vi "sub_tcp_fgv.vi"(7 "cmd":enum16{"ini", "read", "write", "close"}(ring), 8 "error in (no error)":errorcluster caption="error in", 11 "write_data":string) -> (0 "error out":errorcluster, 2 "data_check":bool, 3 "read_data":string)   [LabVIEW 2018]
panel:
  out "byte":u8[](array[numeric])
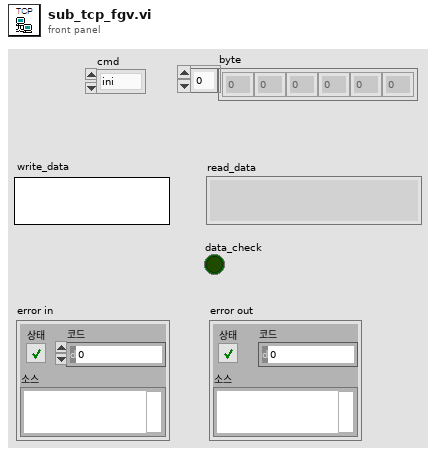
[diagram p1: front panel]
types:
  T1 = enum16{"Standard", "Buffered", "CRLF", "Immediate"}
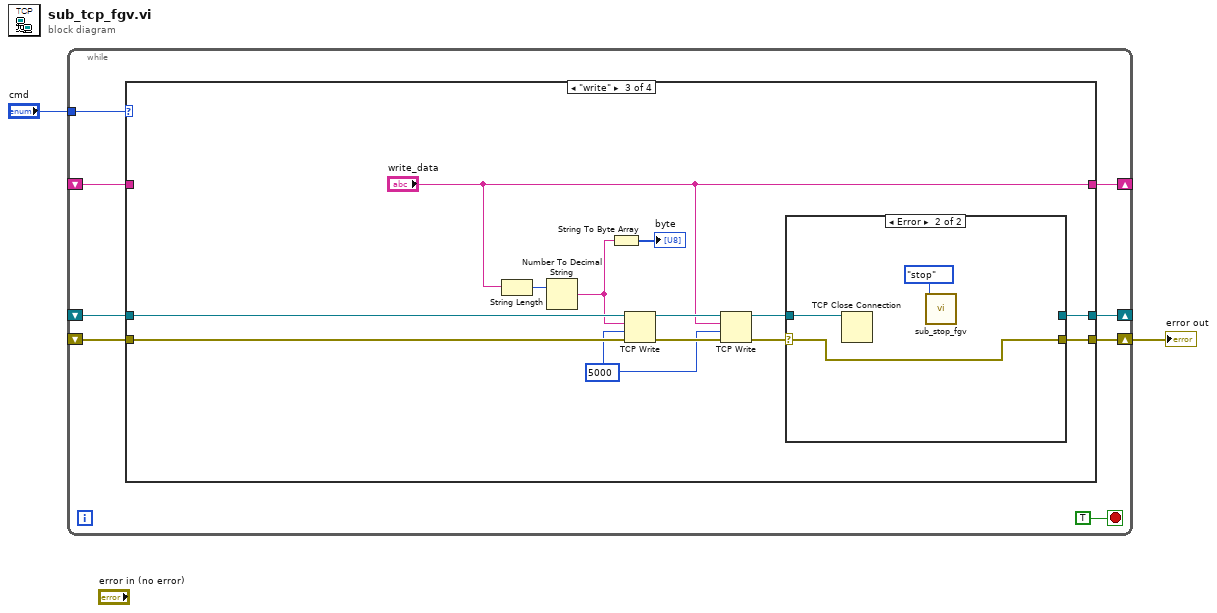
[diagram p0: block diagram]
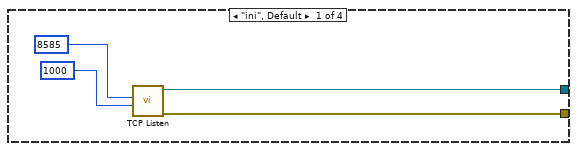
[diagram p2: hidden frame]
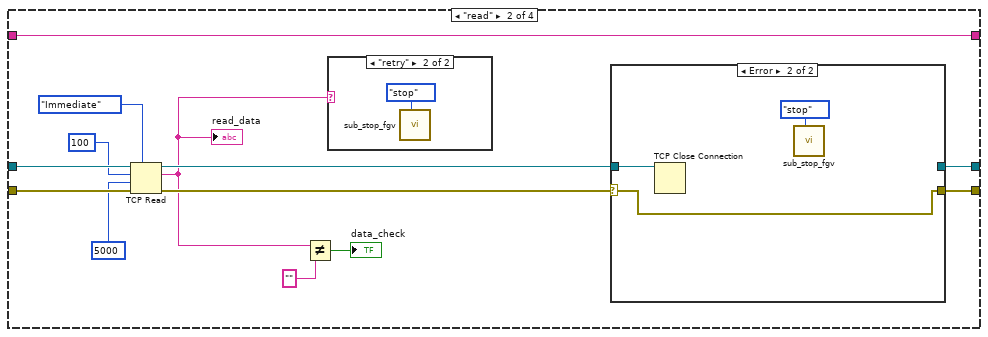
[diagram p3: hidden frame]
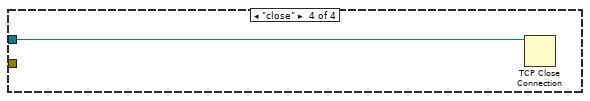
[diagram p7: hidden frame]
diagram:
  n1 = while {
    tunnel: "cmd" -> [w9]
    shift-right: [w7] -> _
    shift-left: _ -> [w6]
    shift-right: [w8] -> w1
    shift-left: _ -> [w5]
    shift-right: [w4] -> _
    shift-left: _ -> [w3]
    stop <- TRUE stop-if-true
    n2 = case shown="\"write\"" w9 {
      tunnel: [w12 w24 w38 _] -> w8
      tunnel: [w11 w25 w39 _] -> w7
      tunnel: w6 -> [_ w27 w44 w52]
      tunnel: w5 -> [_ w26 w45 _]
      tunnel: [_ w18 "write_data" _] -> w4
      tunnel: w3 -> [_ w18 _ _]
      frame "ini", Default {
        n3 = call <vilib>:"TCP Listen.vi"("timeout ms (wait forever: -1)"=1000, "port"=u16 8585) -> ("error out"=w12:errorcluster, "connection ID"=w11:refnum<k5>)  [unwired: 5 in, 3 out]
      }
      frame "read" {
        n4 = TCP Read(connection ID=w27, bytes to read=100 ("읽을 바이트"), error in (no error)=w26, 7:T1."Immediate" ("모드(standard)"), 9:5000 ("타임아웃 ms (25000)")) -> (connection ID out=w19:refnum<k5>, data out=w16:string, error out=w20:errorcluster)
        "read_data" <- w16
        n5 = Not Equal?(x=w16, y="") -> (x != y?=→"data_check":bool)
        n6 = case shown="\"retry\"" w16 {
          frame "거짓", Default {
          }
          frame "retry" {
            n7 = call "sub_stop_fgv.vi"("cmd"=enum16{"ini", "check", "stop"}."stop") -> ()  [unwired: 10 in, 1 out]
          }
        }
        n8 = case shown="Error" w20 {
          selector: w20 -> [w29 w31]
          tunnel: w19 -> [w30 w33]
          tunnel: [w30 _] -> w25
          tunnel: [w29 w31] -> w24
          frame No Error {
          }
          frame Error {
            n9 = TCP Close Connection(connection ID=w33) -> ()  [unwired: 1 in, 3 out]
            n10 = call "sub_stop_fgv.vi"("cmd"=enum16{"ini", "check", "stop"}."stop") -> ()  [unwired: 10 in, 1 out]
          }
        }
      }
      frame "write" {
        w34 = 5000 ("타임아웃 ms (25000)")
        n11 = String Length(string="write_data") -> (length=w42:i32)
        n12 = Number To Decimal String(number=w42) -> (decimal integer string=w36:string)  [unwired: 1 in]
        n13 = String To Byte Array(string=w36) -> (unsigned byte array=→"byte":u8[])
        n14 = TCP Write(connection ID=w44, data in=w36, error in (no error)=w45, 9:w34) -> (connection ID out=w43:refnum<k5>, error out=w46:errorcluster)  [unwired: 1 out]
        n15 = TCP Write(connection ID=w43, data in="write_data", error in (no error)=w46, 9:w34) -> (connection ID out=w40:refnum<k5>, error out=w41:errorcluster)  [unwired: 1 out]
        n16 = case shown="Error" w41 {
          selector: w41 -> [w47 w49]
          tunnel: w40 -> [w48 w51]
          tunnel: [w48 _] -> w39
          tunnel: [w47 w49] -> w38
          frame No Error {
          }
          frame Error {
            n17 = TCP Close Connection(connection ID=w51) -> ()  [unwired: 1 in, 3 out]
            n18 = call "sub_stop_fgv.vi"("cmd"=enum16{"ini", "check", "stop"}."stop") -> ()  [unwired: 10 in, 1 out]
          }
        }
      }
      frame "close" {
        n19 = TCP Close Connection(connection ID=w52) -> ()  [unwired: 1 in, 3 out]
      }
    }
  }
  "error out" <- w1
